vi "Main.vi"() -> ()   [LabVIEW 2019]
doc: "GUI DEMO Wolfgang Zwick, NI Germany"
uses:
  Support/Shared/TypeDefs/Data.ctl
  Support/Shared/TypeDefs/Refs.ctl
  Support/Message Queue/State Name.ctl
  Support/Status/Message Queue/State Name.ctl
  b153a6de-714d-4306-a33b-64952116f927.vi
  a28567d3-7ea8-4969-ae4c-e17c99254f4e.vi
  3415c264-0024-4f32-96ea-a6fdca28e222.vi
  Support/Message Queue/Enqueue (Single).vi
  Support/Status/Status.vi
  Support/Message Queue/Enqueue (Array).vi
  Support/Subpanel Tools/Global - Name of loaded Module.vi
  <vilib>/Platform/browser.llb/Open URL in Default Browser (string).vi
  Support/Status/Message Queue/Reference Queue.vi
  <vilib>/Utility/error.llb/Error Cluster From Error Code.vi
  <vilib>/ErrorRing/Error Ring.xnode
  Support/User Event - Stop/User Event - Stop.lvlib
  Support/Subpanel Tools/Subpanel Tools.lvlib
  Support/UI Tools/UI Tools.lvlib
  Support/Status/Status.lvlib
  Support/Message Queue/Message Queue.lvlib
panel:
  in  "Radio Buttons":enum32{"Acquire", "Explore", "Present"}(radio)
  out "Status Bar":string
  out "Progress Bar":u8(slide) scale=0.0..100.0
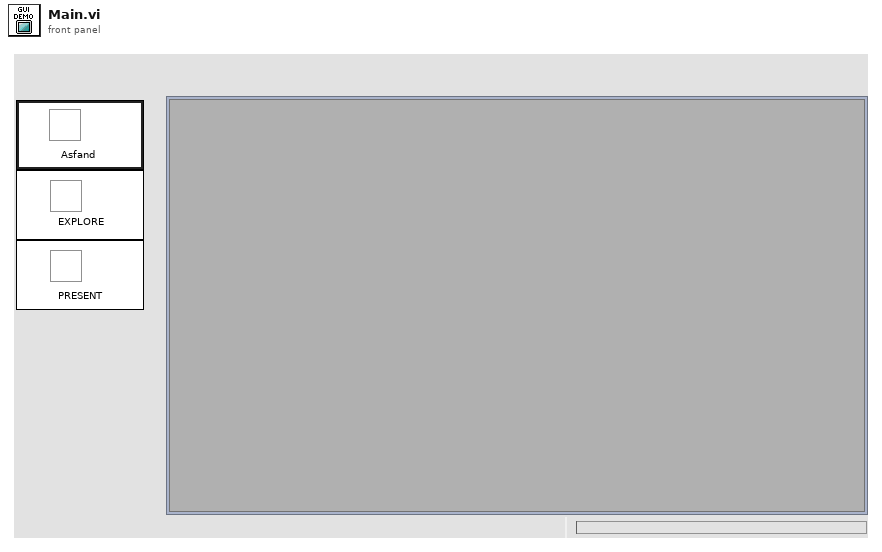
[diagram p1: front panel]
types:
  T1 = typedef "Message Queue.lvlib/State Name.ctl" = enum16{"Default", "Initialize", "Initialize Data", "Initialize Modules", "Initialize Panel", "Close FP", "Open FP", "Initialize Menu", "Mode", "Update Subpanel", "Error", "Open Help", "About", "Open WebResources", "Exit"}
  T2 = typedef "Data.ctl" = cluster{"Refs":T3, "Settings File":path, "ModuleConfig File":path, "Modules":path}
  T3 = typedef "Refs.ctl" = cluster{"VI Refnum":refnum<vi>, "Radio Buttons Ref":refnum<vi>, "Sub Panel Ref":refnum<vi>, "VI Refs":refnum<vi>[]}
  T4 = typedef "Message Queue Ref.ctl" = refnum<queue>
  T5 = enum32{"Invalid", "Standard", "Closed", "Hidden", "Minimized", "Maximized"}
  T6 = typedef "Status.lvlib/State Name.ctl" = enum16{"Initialize", "Update Progress Bar", "Update Status Bar", "Set Cursor Busy", "Unset Cursor Busy", "Error", "Default", "Exit"}
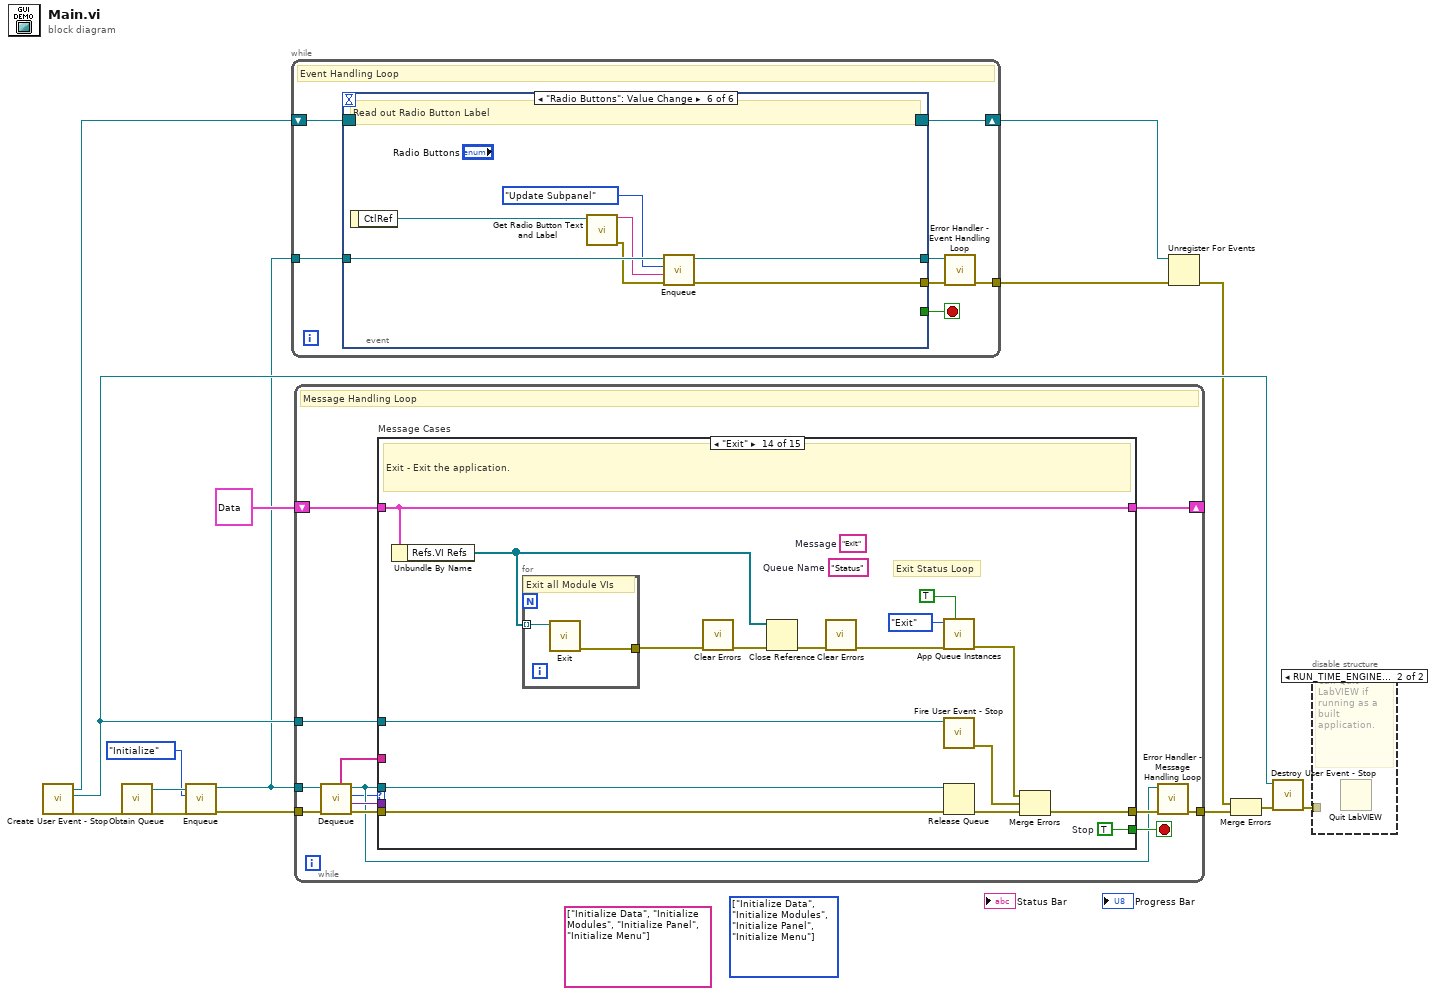
[diagram p0: block diagram]
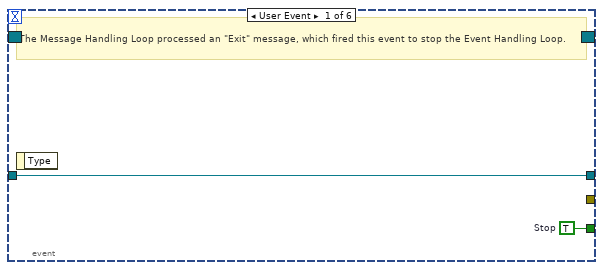
[diagram p3: hidden frame]
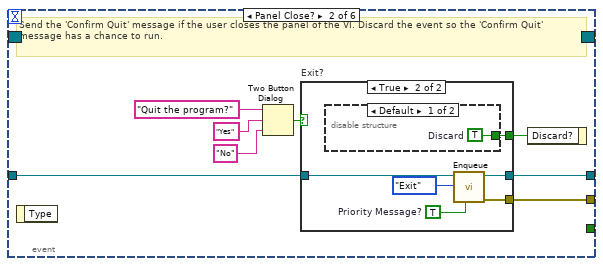
[diagram p4: hidden frame]
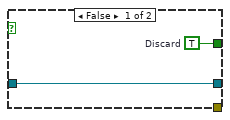
[diagram p5: hidden frame]
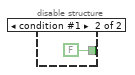
[diagram p6: hidden frame]
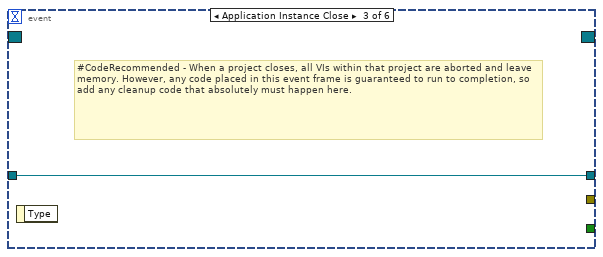
[diagram p7: hidden frame]
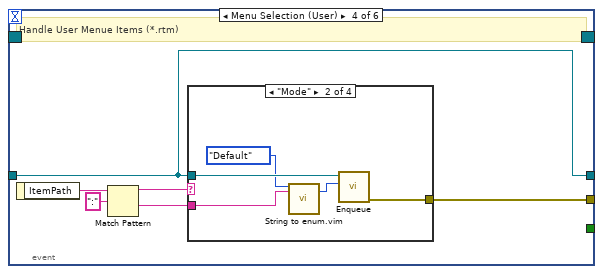
[diagram p8: hidden frame]
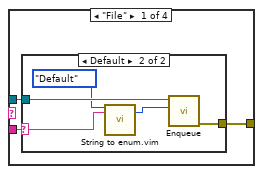
[diagram p9: hidden frame]
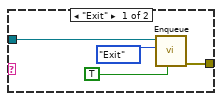
[diagram p10: hidden frame]
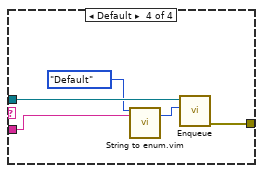
[diagram p12: hidden frame]
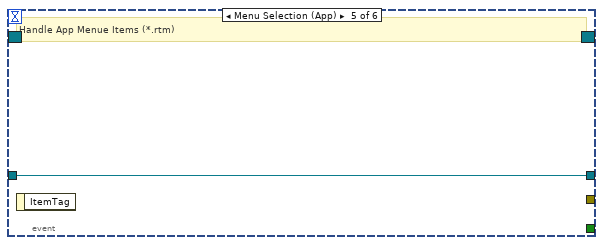
[diagram p13: hidden frame]
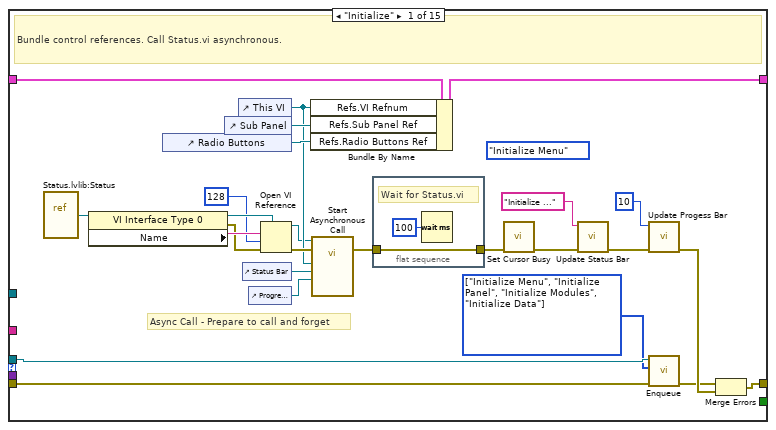
[diagram p14: hidden frame]
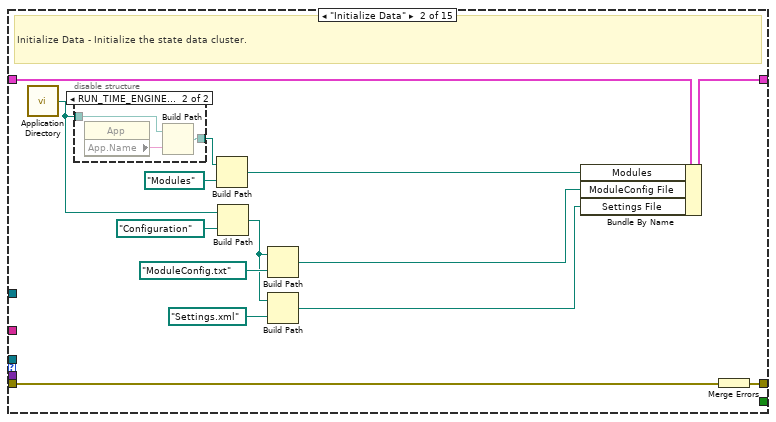
[diagram p15: hidden frame]
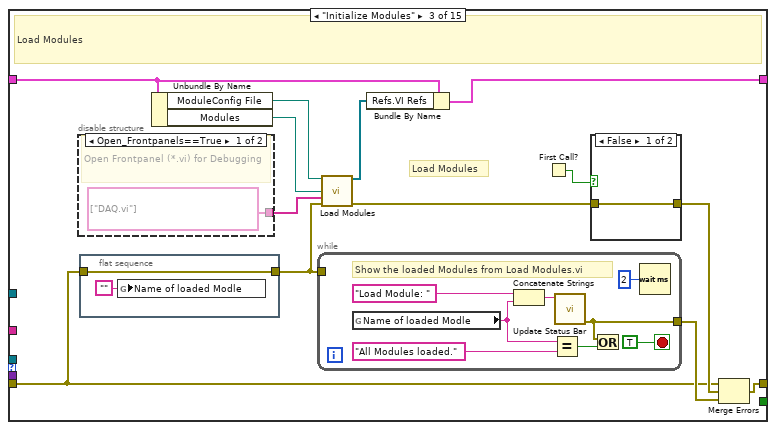
[diagram p17: hidden frame]
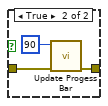
[diagram p18: hidden frame]
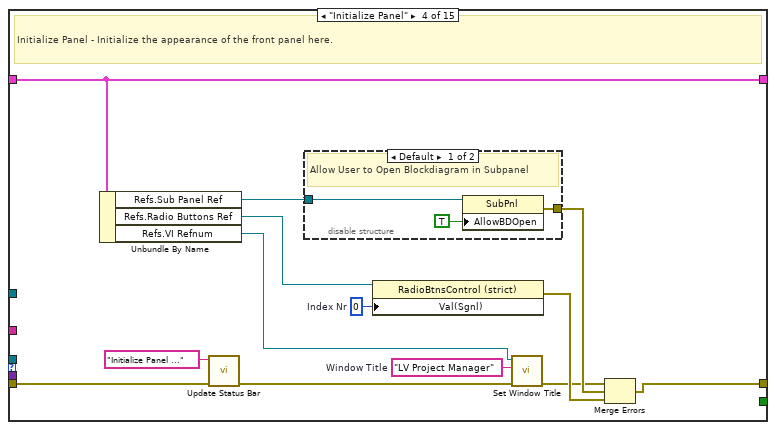
[diagram p20: hidden frame]
diagram:
  (unwired) string[] ["Initialize Data", "Initialize Modules", "Initialize Panel", "Initialize Menu"]
  (unwired) T1[] [enum."Initialize Data", enum."Initialize Modules", enum."Initialize Panel", enum."Initialize Menu"] items=["Default", "Initialize", "Initialize Data", "Initialize Modules", "Initialize Panel", "Close FP", "Open FP", "Initialize Menu", "Mode", "Update Subpanel", "Error", "Open Help", "About", "Open WebResources", "Exit"] ("States")
  n1 = call "Create User Event - Stop.vi"() -> ("error out"=w2:errorcluster, "User Event - Stop"=w13:refnum<user-event>, "Event Registration Refnum Out"=w4:refnum<event-registration>)  [unwired: 9 in]
  n2 = call "Obtain Queue.vi"("error in (no error)"=w2) -> ("error out"=w6:errorcluster, "Message Queue out"=w7:T4)  [unwired: 9 in]
  n3 = call-poly "Enqueue.vi"("error in (no error)"=w6, "States"=State_Name."Initialize", "Message Queue"=w7) -> ("error out"=w5:errorcluster, "dup Message Queue"=w3:T4)  [unwired: 7 in]
  n4 = while {
    tunnel: w3 -> [w22]
    shift-right: [w20] -> w11
    shift-left: w4 -> [w21]
    tunnel: [w16] -> w8
    stop <- w18 stop-if-true
    # "Event Handling Loop"
    n5 = event shown="[5] \"Radio Buttons\": Value Change" {
      selector: w21 -> [_ _ _ _ _ _]
      dyn-events: [_ _ _ _ _ _] -> w20
      timeout: _ -> [_ _ _ _ _ _]
      tunnel: [w23 _ _ _ _ _] -> w18
      tunnel: w22 -> [w24 w32 w43 w44 w72 w79]
      tunnel: [_ w31 _ w49 _ w76] -> w19
      tunnel: [w24 w30 w43 w44 w72 w78] -> w17
      event User Event {
        w23 = TRUE  # Stop
        # "The Message Handling Loop processed an \"Exit\" message, which fired this event to stop the Event Handling Loop."
        n6 = event-data() -> ()  [unwired: 1 in, 1 out]
      }
      event Panel Close? {
        # "Send the 'Confirm Quit' message if the user closes the panel of the VI. Discard the event so the 'Confirm Quit' message has a chance to run."
        n7 = event-data() -> ()  [unwired: 1 in, 1 out]
        n8 = Two Button Dialog(message="Quit the program?", 1:"No" ("F button name (\"Cancel\")"), 2:"Yes" ("T button name (\"OK\")")) -> (T button?=w26:bool)
        n9 = case "Exit?" shown="True" w26 {
          tunnel: w32 -> [w34 w40]
          tunnel: [_ w39] -> w31
          tunnel: [w34 w38] -> w30
          tunnel: [w33 w36] -> w25
          frame False {
            w33 = TRUE  # Discard
          }
          frame True {
            w37 = TRUE  # Priority Message?
            n10 = disable-structure shown="Default" {
              disable-tunnel: [w41 FALSE ("Discard")] -> w36
              frame condition #0 (active) {
                w41 = TRUE  # Discard
              }
              frame condition #1 {
              }
            }
            n11 = call-poly "Enqueue.vi"("Priority Message? Array"=w37, "States"=State_Name."Exit", "Message Queue"=w40) -> ("error out"=w39:errorcluster, "dup Message Queue"=w38:T4)  [unwired: 7 in]
          }
        }
        n12 = event-data("Discard?"=w25) -> ()  [unwired: 1 in, 1 out]
      }
      event Application Instance Close {
        # "#CodeRecommended - When a project closes, all VIs within that project are aborted and leave memory. However, any code placed in this event frame is guaranteed to run to completion, so add any cleanup code that absolutely must happen here."
        n13 = event-data() -> ()  [unwired: 1 in, 1 out]
      }
      event Menu Selection (User) {
        # "Handle User Menue Items (*.rtm)"
        n14 = event-data() -> ("ItemPath"=w48:string)  [unwired: 1 in]
        n15 = Match Pattern(string=w48, regular expression=":") -> (before substring=w46:string, after substring=w45:string)  [unwired: 1 in, 2 out]
        n16 = case shown="\"Mode\"" w46 {
          tunnel: w44 -> [w52 w66 _ w70]
          tunnel: [w51 w65 _ w69] -> w49
          tunnel: w45 -> [w50 w62 _ w68]
          frame "File" {
            n17 = case shown="Default" w50 {
              selector: w50 -> [_ w58]
              tunnel: w52 -> [w56 w61]
              tunnel: [w55 w60] -> w51
              frame "Exit" {
                n18 = call-poly "Enqueue.vi"("Priority Message? Array"=TRUE ("Priority Message? (F)"), "States"=State_Name."Exit", "Message Queue"=w56) -> ("error out"=w55:errorcluster)  [unwired: 7 in, 1 out]
              }
              frame Default {
                n19 = call "String to enum.vim"("Enum"=State_Name."Default" ("States"), "Item Name"=w58) -> ("Enum Selected"=w57:u16)  [unwired: 15 in, 2 out]
                n20 = call-poly "Enqueue.vi"("States"=w57, "Message Queue"=w61) -> ("error out"=w60:errorcluster)  [unwired: 8 in, 1 out]
              }
            }
          }
          frame "Mode" {
            n21 = call "String to enum.vim"("Enum"=State_Name."Default" ("States"), "Item Name"=w62) -> ("Enum Selected"=w63:u16)  [unwired: 15 in, 2 out]
            n22 = call-poly "Enqueue.vi"("States"=w63, "Message Queue"=w66) -> ("error out"=w65:errorcluster)  [unwired: 8 in, 1 out]
          }
          frame "Options" {
          }
          frame Default {
            n23 = call "String to enum.vim"("Enum"=State_Name."Default" ("States"), "Item Name"=w68) -> ("Enum Selected"=w71:u16)  [unwired: 15 in, 2 out]
            n24 = call-poly "Enqueue.vi"("States"=w71, "Message Queue"=w70) -> ("error out"=w69:errorcluster)  [unwired: 8 in, 1 out]
          }
        }
      }
      event Menu Selection (App) {
        # "Handle App Menue Items (*.rtm)"
        n25 = event-data() -> ()  [unwired: 1 in, 1 out]
      }
      event "Radio Buttons": Value Change {
        # "Read out Radio Button Label"
        n26 = event-data() -> ("CtlRef"=w75:refnum<vi>)  [unwired: 1 in]
        n27 = call "Get Radio Button Text and Label.vi"("error in"=w75) -> ("selected Buton.Text"=w73:string, "filenames out"=w77:errorcluster)  [unwired: 10 in, 3 out]
        n28 = call-poly "Enqueue.vi"("error in (no error)"=w77, "Message Data Array"=w73, "States"=State_Name."Update Subpanel", "Message Queue"=w79) -> ("error out"=w76:errorcluster, "dup Message Queue"=w78:T4)  [unwired: 6 in]
      }
    }
    n29 = call "Error Handler - Event Handling Loop.vi"("error in (no error)"=w19, "Message Queue"=w17) -> ("dup error in"=w16:errorcluster)  [unwired: 8 in, 1 out]
  }
  n30 = while {
    tunnel: w3 -> [w83]
    shift-right: [w91] -> _
    shift-left: T2 {"Refs"={"VI Refnum"=refnum, "Radio Buttons Ref"=refnum, "Sub Panel Ref"=refnum, "VI Refs"=[]}, "Settings File"=path "", "ModuleConfig File"=path "", "Modules"=path ""} ("Data Cluster") -> [w92]
    tunnel: w13 -> [w89]
    tunnel: w5 -> [w88]
    tunnel: [w84] -> w15
    stop <- w90 stop-if-true
    # "Message Handling Loop"
    n31 = call "Dequeue.vi"("error in (no error)"=w88, "Message Queue"=w83) -> ("error out"=w87:errorcluster, "Message Data"=w86:variant, "State"=w81:T1, "dup Message Queue"=w82:refnum<queue>, "Call Chain"=w80:string[])  [unwired: 4 in, 1 out]
    n32 = case "Message Cases" shown="\"Exit\"" w81 {
      selector: w81 -> [_ _ _ _ _ _ _ _ _ _ _ _ _ _ w300]
      tunnel: w82 -> [w118 _ _ _ _ _ _ _ _ w242 _ _ _ w297 _]
      tunnel: w87 -> [w99 w127 w141 w170 w199 w213 w224 w230 w235 w249 w251 w276 w280 w290 _]
      tunnel: [w114 w134 w151 w179 w204 w215 w226 w229 w234 w243 w252 w275 w279 w294 w301] -> w85
      tunnel: w92 -> [w117 w133 w148 w178 w203 w214 w225 w231 w236 w248 w253 w277 w281 w291 w302]
      tunnel: [w113 w132 w150 w178 w203 w214 w225 w231 w236 w248 w253 w277 w281 w291 w302] -> w91
      tunnel: [_ _ _ _ _ _ _ _ _ _ _ _ _ w296 _] -> w90
      tunnel: w86 -> [_ _ _ _ _ w209 w223 _ _ w247 _ _ _ _ _]
      tunnel: w89 -> [_ _ _ _ _ _ _ _ _ _ _ _ _ w293 _]
      tunnel: w80 -> [_ _ _ _ _ _ _ _ _ _ _ _ _ _ _]
      frame "Initialize" {
        (unwired) State_Name."Initialize Menu" ("State")
        w95 = T1[] [enum."Initialize Menu", enum."Initialize Panel", enum."Initialize Modules", enum."Initialize Data"] items=["Default", "Initialize", "Initialize Data", "Initialize Modules", "Initialize Panel", "Close FP", "Open FP", "Initialize Menu", "Mode", "Update Subpanel", "Error", "Open Help", "About", "Open WebResources", "Exit"] ("Array")
        # "Async Call - Prepare to call and forget"
        # "Bundle control references. Call Status.vi asynchronous."
        n33 = vi-ref "Status.lvlib:Status.vi"() -> (w105:refnum<vi>)
        n34 = property class="VI Interface Type 0"(reference=w105) -> (reference out=w109:refnum<vi>, error out=w107:errorcluster, "Name"=w110:string)  [unwired: 1 in]
        n35 = control-ref of="Radio Buttons"() -> (w115:refnum<vi>)
        n36 = control-ref of="Sub Panel"() -> (w116:refnum<vi>)
        n37 = control-ref of="This VI"() -> (w104:refnum<vi>)
        n38 = control-ref of="Status Bar"() -> (w103:refnum<vi>)
        n39 = control-ref of="Progress Bar"() -> (w102:refnum<vi>)
        n40 = Open VI Reference(type specifier VI Refnum (for type only)=w109, vi path=w110, options=128, error in (no error)=w107) -> (vi reference=w93:refnum<vi>, error out=w106:errorcluster)  [unwired: 2 in]
        n41 = Bundle By Name(cluster=w117, "Refs.VI Refnum"=w104, "Refs.Sub Panel Ref"=w116, "Refs.Radio Buttons Ref"=w115) -> (w113:T2)
        n42 = call-by-ref "Start Asynchronous Call"(reference=w93, error in=w106, "Progress Bar"=w102, "Status Bar"=w103, "VI Refnum"=w104) -> (error out=w97:errorcluster)  [unwired: 8 in, 2 out]
        n43 = flat-sequence {
          tunnel: w97 -> [w119]
          tunnel: [w119] -> w96
          frame #0 {
            # "Wait for Status.vi"
            n44 = Wait (ms)(milliseconds to wait=u32 100) -> ()  [unwired: 1 out]
          }
        }
        n45 = call "Set Cursor Busy.vi"("error in (no error)"=w96) -> ("error out"=w112:errorcluster)  [unwired: 10 in]
        n46 = call "Update Status Bar.vi"("error in (no error)"=w112, "Status Bar"="Initialize ...") -> ("error out"=w101:errorcluster)  [unwired: 9 in]
        n47 = call "Update Progess Bar.vi"("error in (no error)"=w101, "Progess Bar"=u8 10) -> ("error out"=w100:errorcluster)  [unwired: 9 in]
        n48 = call-poly "Enqueue.vi"("error in (no error)"=w99, "States"=w95, "Message Queue"=w118) -> ("error out"=w94:errorcluster)  [unwired: 7 in, 1 out]
        n49 = Merge Errors(w94, w100) -> (w114:errorcluster)
      }
      frame "Initialize Data" {
        # "Initialize Data - Initialize the state data cluster."
        n50 = call <vilib>:"Application Directory.vi"() -> ("Application Directory"=w124:path)
        n51 = disable-structure shown="RUN_TIME_ENGINE==True" {
          disable-tunnel: w124 -> [w135 w138]
          disable-tunnel: [w135 w137] -> w125
          frame condition #0 (active) {
          }
          frame condition #1 {
            n52 = property class="App"() -> ("App.Name"=w136:string)  [unwired: 2 in, 2 out]
            n53 = Build Path(base path=w138, name or relative path=w136) -> (appended path=w137:path)
          }
        }
        n54 = Build Path(base path=w125, name or relative path=path "Modules" ("File Path (*.XML)")) -> (appended path=w126:path)
        n55 = Build Path(base path=w124, name or relative path=path "Configuration" ("File Path (*.XML)")) -> (appended path=w123:path)
        n56 = Build Path(base path=w123, name or relative path=path "ModuleConfig.txt" ("File Path (*.XML)")) -> (appended path=w122:path)
        n57 = Build Path(base path=w123, name or relative path=path "Settings.xml" ("File Path (*.XML)")) -> (appended path=w121:path)
        n58 = Bundle By Name(cluster=w133, "Modules"=w126, "ModuleConfig File"=w122, "Settings File"=w121) -> (w132:T2)
        n59 = Merge Errors(w127) -> (w134:errorcluster)
      }
      frame "Initialize Modules" {
        # "Load Modules"
        # "Load Modules"
        n60 = disable-structure shown="Open_Frontpanels==True" {
          disable-tunnel: [string[] ["DAQ.vi"] ("Open Frontpanel (*.vi)") _] -> w143
          frame condition #0 {
            # "Open Frontpanel (*.vi) for Debugging"
          }
          frame condition #1 (active) {
          }
        }
        n61 = flat-sequence {
          tunnel: w141 -> [w156]
          tunnel: [w156] -> w140
          frame #0 {
            n62 = global write "Global - Name of loaded Module.vi" "Name of loaded Modle"("") -> ()
          }
        }
        n63 = Unbundle By Name(w148) -> ("ModuleConfig File"=w147:path, "Modules"=w146:path)
        n64 = while {
          tunnel: [w164] -> w142
          tunnel: w140 -> [_]
          stop <- TRUE stop-if-true
          # "Show the loaded Modules from Load Modules.vi"
          n65 = global read "Global - Name of loaded Module.vi" "Name of loaded Modle"() -> (w159:string)
          n66 = Concatenate Strings("Load Module: " ("string"), w159) -> (w161:string)
          n67 = Equal?(x=w159, y="All Modules loaded.") -> (x = y?=w165:bool)
          n68 = call "Update Status Bar.vi"("Status Bar"=w161) -> ("error out"=w164:errorcluster)  [unwired: 10 in]
          n69 = Or(x=w164, y=w165) -> ()  [unwired: 1 out]
          n70 = Wait (ms)(milliseconds to wait=u32 2) -> ()  [unwired: 1 out]
        }
        n71 = call "Load Modules.vi"("Configuration folder"=w147, "Modules folder"=w146, "Open Frontpanel (VI Namei)"=w143, "error in (no error)"=w140) -> ("VI Refs Out"=w149:refnum<vi>[], "error out"=w145:errorcluster)  [unwired: 9 in, 1 out]
        n72 = Bundle By Name(cluster=w148, "Refs.VI Refs"=w149) -> (w150:T2)
        n73 = First Call?() -> (First Call?: T/F=w139:bool)
        n74 = case shown="False" w139 {
          tunnel: w145 -> [w152 w154]
          tunnel: [w152 w153] -> w144
          frame False {
          }
          frame True {
            n75 = call "Update Progess Bar.vi"("error in (no error)"=w154, "Progess Bar"=u8 90 ("Progress Bar")) -> ("error out"=w153:errorcluster)  [unwired: 9 in]
          }
        }
        n76 = Merge Errors(w141, w144, w142) -> (w151:errorcluster)
      }
      frame "Initialize Panel" {
        w171 = "LV Project Manager"  # Window Title
        w167 = u32 0  # Index Nr
        # "Initialize Panel - Initialize the appearance of the front panel here."
        n77 = Unbundle By Name(w178) -> ("Refs.Sub Panel Ref"=w177:refnum<vi>, "Refs.Radio Buttons Ref"=w175:refnum<vi>, "Refs.VI Refnum"=w172:refnum<vi>)
        n78 = call "Update Status Bar.vi"("error in (no error)"=w170, "Status Bar"="Initialize Panel ...") -> ("error out"=w169:errorcluster)  [unwired: 9 in]
        n79 = disable-structure shown="Default" {
          disable-tunnel: w177 -> [w181 w185]
          disable-tunnel: [w180 w184] -> w176
          frame condition #0 (active) {
            # "Allow User to Open Blockdiagram in Subpanel"
            n80 = property class="SubPnl"(reference=w181, "AllowBDOpen"=TRUE ("Allow User to Open Diagram")) -> (error out=w180:errorcluster)  [unwired: 1 in, 1 out]
          }
          frame condition #1 {
            n81 = property class="SubPnl"(reference=w185, "AllowBDOpen"=FALSE ("Allow User to Open Diagram")) -> (error out=w184:errorcluster)  [unwired: 1 in, 1 out]
          }
        }
        n82 = property class="RadioBtnsControl (strict)"(reference=w175, "Val(Sgnl)"=w167) -> (error out=w174:errorcluster)  [unwired: 1 in, 1 out]
        n83 = call "Set Window Title.vi"("error in (no error)"=w169, "Window Title"=w171, "VI Refnum In"=w172) -> ("error out"=w173:errorcluster)  [unwired: 7 in, 1 out]
        n84 = Merge Errors(w173, w176, w174) -> (w179:errorcluster)
      }
      frame "Initialize Menu" {
        w202 = "Mode"  # menu tag
        # "Initialize Menue - Set Status and Progress Bar, create menu tag 'Mode' from Radio Button Labels"
        n85 = Unbundle By Name(w203) -> ("Refs.Radio Buttons Ref"=w197:refnum<vi>)
        n86 = call "Update Status Bar.vi"("Status Bar"="Initialize Panel ...") -> ("error out"=w186:errorcluster)  [unwired: 10 in]
        n87 = call "Get Radio Button Text and Label.vi"("error in"=w197, "filenames in"=w186) -> ("Button.Text []"=w198:string[], "filenames out"=w200:errorcluster)  [unwired: 9 in, 3 out]
        n88 = Current VI's Menubar() -> (w201:refnum<k9>)
        n89 = Insert Menu Items(5:w202, 6:w200, 7:w198, 8:w198, 9:w201) -> (0:w196:errorcluster)  [unwired: 1 in, 2 out]
        n90 = call "Update Progess Bar.vi"("error in (no error)"=w196, "Progess Bar"=u8 100 ("Progress Bar")) -> ("error out"=w194:errorcluster)  [unwired: 9 in]
        n91 = flat-sequence {
          tunnel: w194 -> [w205]
          tunnel: [w205] -> w193
          frame #0 {
            n92 = Wait (ms)(milliseconds to wait=u32 200) -> ()  [unwired: 1 out]
          }
        }
        n93 = call "Update Progess Bar.vi"("error in (no error)"=w193, "Progess Bar"=u8 0) -> ("error out"=w191:errorcluster)  [unwired: 9 in]
        n94 = call "Update Status Bar.vi"("error in (no error)"=w191, "Status Bar"="") -> ("error out"=w190:errorcluster)  [unwired: 9 in]
        n95 = call "Unset Cursor Busy.vi"("error in (no error)"=w190) -> ("error out"=w189:errorcluster)  [unwired: 10 in]
        n96 = Merge Errors(w199, w189) -> (w204:errorcluster)
      }
      frame "Mode" {
        # "Mode - Change"
        n97 = Unbundle By Name(w214) -> ("Refs.Radio Buttons Ref"=w207:refnum<vi>)
        n98 = Variant To Data(error in=w213, type="", Variant=w209) -> (data=w211:string, error out=w212:errorcluster)
        n99 = call "Set Radio Button (Value Sgnl).vi"("Radio Buttons Ref In"=w207, "Radio Button Text"=w211, "error in (no error)"=w212) -> ("error out"=w208:errorcluster)  [unwired: 11 in, 1 out]
        n100 = Merge Errors(w208) -> (w215:errorcluster)
      }
      frame "Update Subpanel" {
        # "Update Suppanel and Update Status Bar"
        n101 = Variant To Data(error in=w224, type="", Variant=w223) -> (data=w219:string, error out=w218:errorcluster)
        n102 = Unbundle By Name(w225) -> ("Refs.Sub Panel Ref"=w221:refnum<vi>, "Refs.VI Refs"=w220:refnum<vi>[])
        n103 = call "Load to Subpanel.vi"("Sub Panel Ref In"=w221, "VI Refs In"=w220, "Module Name In"=w219, "error in (no error)"=w218) -> ("error out"=w217:errorcluster)  [unwired: 8 in, 3 out]
        n104 = call <vilib>:"Clear Errors.vi"("error in (no error)"=w217) -> ("error out"=w216:errorcluster)  [unwired: 5 in, 1 out]
        n105 = Merge Errors(w216) -> (w226:errorcluster)
      }
      frame "Close FP" {
        n106 = invoke class="VI" method="FP.Open"(error in=w230, "Activate"=TRUE ("Activate?"), "State"=T5."Hidden") -> (error out=w229:errorcluster)  [unwired: 2 in, 4 out]
      }
      frame "Open FP" {
        n107 = invoke class="VI" method="FP.Open"(error in=w235, "Activate"=TRUE ("Activate?"), "State"=T5."Standard") -> (error out=w234:errorcluster)  [unwired: 2 in, 4 out]
      }
      frame "Error" {
        w241 = TRUE  # Priority Message? (F)
        # "Error - Check the error message data and respond accordingly. This message is sent by the \"Error Handler\" VIs at the end of each loop in this application."
        n108 = call-poly "Enqueue.vi"("Priority Message? Array"=w241, "States"=State_Name."Exit", "Message Queue"=w242) -> ("error out"=w244:errorcluster)  [unwired: 7 in, 1 out]
        n109 = Variant To Data(error in=w249, type=errorcluster {"status"=FALSE, "code"=0, "source"=""} ("error constant"), Variant=w247) -> (data=w245:errorcluster, error out=w239:errorcluster)
        n110 = call <vilib>:"Simple Error Handler.vi"("error in (no error)"=w245) -> ("message"=w240:string)  [unwired: 4 in, 4 out]
        n111 = call "Update Status Bar.vi"("error in (no error)"=w239, "Status Bar"=w240) -> ("error out"=w238:errorcluster)  [unwired: 9 in]
        n112 = Merge Errors(w244, w238) -> (w243:errorcluster)
      }
      frame "Open Help" {
        # "Open Help"
        n113 = disable-structure shown="Enabled" {
          disable-tunnel: w251 -> [w257 w263]
          disable-tunnel: [w256 w262] -> w250
          frame Disabled {
            w254 = "lvdialog.chm"  # CHM or HLP filename (lvdialog.chm)
            w255 = ""  # HTML filename
            n114 = call "_LaunchHelp.vi"("error in (no error)"=w257, "CHM or HLP filename (lvdialog.chm)"=w254, "HTML filename"=w255) -> ("error out"=w256:errorcluster)  [unwired: 4 in]
          }
          frame Enabled {
            n115 = Current VI's Path() -> (path=w261:path)
            n116 = Strip Path(path=w261) -> (stripped path=w259:path)  [unwired: 1 out]
            n117 = disable-structure shown="RUN_TIME_ENGINE==True" {
              disable-tunnel: [w266 w269] -> w258
              disable-tunnel: path "GUI Demo.pdf" ("Application Directory") -> [w264 w270]
              disable-tunnel: w259 -> [w267 w274]
              frame condition #0 (active) {
                n118 = Build Path(base path=w267, name or relative path=path "Documentation/GUI Demo Documentation" ("Application Directory")) -> (appended path=w265:path)
                n119 = Build Path(base path=w265, name or relative path=w264) -> (appended path=w266:path)
              }
              frame condition #1 {
                n120 = Strip Path(path=w274) -> (stripped path=w271:path)  [unwired: 1 out]
                n121 = Build Path(base path=w271, name or relative path=path "Documentation" ("Application Directory")) -> (appended path=w272:path)
                n122 = Build Path(base path=w272, name or relative path=w270) -> (appended path=w269:path)
              }
            }
            n123 = call <vilib>:"Show in File System.vi"("error in (no error)"=w263, "file or directory path"=w258) -> ("error out"=w262:errorcluster)  [unwired: 9 in]
          }
        }
        n124 = Merge Errors(w250) -> (w252:errorcluster)
      }
      frame "About" {
        # "Open About Dialog"
        n125 = call "About Dialog.vi"("error in (no error)"=w276) -> ("error out"=w275:errorcluster)  [unwired: 10 in]
      }
      frame "Open WebResources" {
        w278 = "https://www.ni.com"  # URL
        n126 = call-poly <vilib>:"Open URL in Default Browser.vi"("error in (no error)"=w280, "URL"=w278) -> ("error out"=w279:errorcluster)  [unwired: 4 in, 1 out]
      }
      frame "Exit" {
        (unwired) "Status"  # Queue Name
        (unwired) "Exit"  # Message
        w296 = TRUE  # Stop
        # "Exit Status Loop"
        # "Exit - Exit the application."
        n127 = Unbundle By Name(w291) -> ("Refs.VI Refs"=w285:refnum<vi>[])
        n128 = for {
          tunnel: w285 -> [w299] mode=indexing
          tunnel: [w298] -> w284
          # "Exit all Module VIs"
          n129 = call "Exit.vi"("VI Refnum"=w299) -> ("error out"=w298:errorcluster)  [unwired: 10 in]
        }
        n130 = call <vilib>:"Clear Errors.vi"("error in (no error)"=w284) -> ("error out"=w283:errorcluster)  [unwired: 5 in, 1 out]
        n131 = Close Reference(reference=w285, error in (no error)=w283) -> (error out=w288:errorcluster)
        n132 = call <vilib>:"Clear Errors.vi"("error in (no error)"=w288) -> ("error out"=w286:errorcluster)  [unwired: 5 in, 1 out]
        n133 = call-poly "App Queue Instances.vi"("Priority Message? (F)"=TRUE, "error in (no error)"=w286, "Tasks"=State_Name."Exit") -> ("error out"=w289:errorcluster)  [unwired: 8 in]
        n134 = call "Fire User Event - Stop.vi"("User Event - Stop"=w293) -> ("error out"=w292:errorcluster)  [unwired: 10 in]
        n135 = Release Queue(queue=w297, error in (no error)=w290) -> (error out=w295:errorcluster)  [unwired: 1 in, 2 out]
        n136 = Merge Errors(w289, w292, w295) -> (w294:errorcluster)
      }
      frame Default {
        # "'Default' case only runs if there is a message that isn't defined in any of the other cases.  Output a programming error."
        n137 = xnode "Error Ring"("parameter 0"=w300) -> ("error out"=w301:errorcluster)
      }
    }
    n138 = call "Error Handler - Message Handling Loop.vi"("error in (no error)"=w85, "Message Queue"=w82) -> ("dup error in"=w84:errorcluster)  [unwired: 8 in, 1 out]
  }
  n139 = Unregister For Events(event registration refnum=w11, error in=w8) -> (error out=w12:errorcluster)
  n140 = Merge Errors(w12, w15) -> (w14:errorcluster)
  n141 = call "Destroy User Event - Stop.vi"("error in (no error)"=w14, "User Event - Stop"=w13) -> ("error out"=w9:errorcluster)  [unwired: 9 in]
  n142 = disable-structure shown="RUN_TIME_ENGINE==True" {
    disable-tunnel: w9 -> [_ _]
    frame condition #0 (active) {
    }
    frame condition #1 {
      # "Call Quit LabVIEW if running as a built application."
      n143 = Quit LabVIEW() -> ()  [unwired: 1 in]
    }
  }
